vi "ObtainMsgQueue.vi"(8 "ErrorArray":errorcluster[](array[cluster])) -> (0 "ErrorArray":errorcluster[](array[cluster]), 3 "QueRef":T1)   [LabVIEW 2014, in "Framework.lvlib"]
uses:
  Framework.lvlib
  Typedef/QueRef.ctl
  Typedef/MsgQueue.ctl
  <userlib>/NIST/NISTErrorLib/NISTErrorLib.lvlib
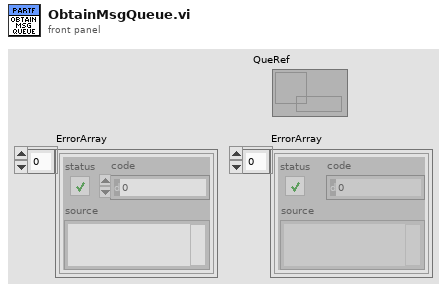
[diagram p1: front panel]
types:
  T1 = typedef "Framework.lvlib/QueRef.ctl" = refnum<queue>
  T2 = typedef "Framework.lvlib/MsgQueue.ctl" = cluster{"Msg":string, "Data":variant}
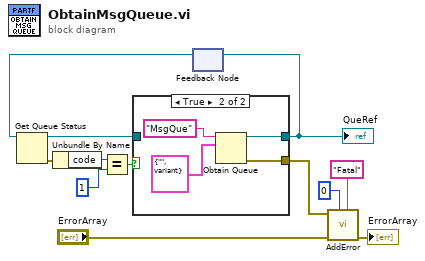
[diagram p0: block diagram]
diagram:
  n1 = feedback #1() -> (w6:refnum<queue>)  [unwired: 1 in]
  n2 = Get Queue Status(queue=w6) -> (queue out=w5:refnum<queue>, error out=w4:errorcluster)  [unwired: 2 in, 6 out]
  n3 = Unbundle By Name(w4) -> ("code"=w2:i32)
  n4 = Equal?(x=w2, y=1) -> (x = y?=w3:bool)
  n5 = case shown="True" w3 {
    tunnel: [w13 w15] -> w12
    tunnel: w5 -> [w13 _]
    tunnel: [_ w14] -> w11
    frame False {
    }
    frame True {
      n6 = Obtain Queue(name (unnamed)="MsgQue", element data type=T2 {"Msg"="", "Data"=variant} ("MsgQueue")) -> (queue out=w15:refnum<queue>, error out=w14:errorcluster)  [unwired: 3 in, 1 out]
    }
  }
  "QueRef" <- w12
  n7 = feedback-in #1(w12) -> ()
  n8 = call <userlib>:"AddError.vi"("Severity"="Fatal", "Priority"=u8 0, "ErrorArray"="ErrorArray", "error in (no error)"=w11) -> ("ErrorArray"=→"ErrorArray":errorcluster[])  [unwired: 6 in, 1 out]
